vi "LinearSystemId_IdentifyDriveTrainSystem.vi"(8 "kAAngular":dbl, 9 "kVAngular":dbl, 10 "kALinear":dbl, 11 "kVLinear":dbl) -> (0 "Size Coerced":bool, 3 "Linearsystem":T1)   [LabVIEW 2019, in "Trajectory_Library.lvlib"]
doc: "Identify a standard differential drive drivetrain, given the drivetrain's kV and kA in both linear (volts/(meter/sec) and volts/(meter/sec^2)) and angular (volts/(meter/sec) and volts/(meter/sec^2)) cases. This can be found using frc-characterization. The linear system is defined as follows:\n\n - states\n - left velocity (m/s)\n - right velocity (m/s)\n - inputs\n - left voltage (volts)\n - right voltage(volts)\n - outputs\n - left velocity (m/s)\n - right velocity (m/s)\n\nInputs: \n - kVLinear -- The linear velocity gain, volts per (meter per second).\n - kALinear -- The linear acceleration gain, volts per (meter per second squared).\n - kVAngular -- The angular velocity gain, volts per (meter per second).\n - kAAngular -- The angular acceleration gain, volts per (meter per second squared).\n\nOutputs:\n - LinearSystem -- A LinearSystem representing the given characterized constants.\n - SizeCoerced -- A boolean indicating an error occured creating the system. A value of TRUE indicates an error.\n\nAdditional information\n https://github.com/wpilibsuite/frc-characterization"
uses:
  Trajectory_Library.lvlib
  TypeDef/LINEAR_SYSTEM.ctl
  <vilib>/Analysis/Matrix/Datatypes/RealMatrix.ctl
  MatrixHelper_CoerceSize.vi
  <vilib>/Analysis/Matrix/NI_Matrix.lvlib
panel:
  # "<States,States>"
  # "<States,Inputs>"
  # "<Outputs,States>"
  # "<Outputs,Inputs>"
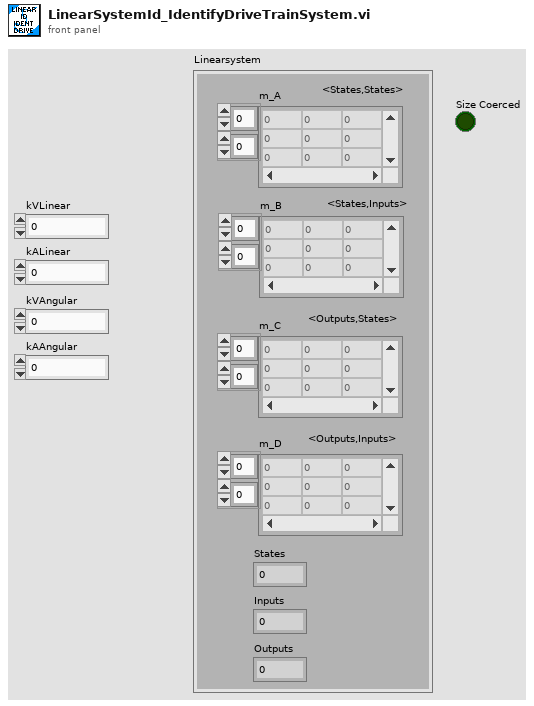
[diagram p1: front panel]
types:
  T1 = typedef "Trajectory_Library.lvlib/LINEAR_SYSTEM.ctl" = cluster{"m_A":T2, "m_B":T2, "m_C":T2, "m_D":T2, "States":i32, "Inputs":i32, "Outputs":i32}
  T2 = typedef "NI_Matrix.lvlib/RealMatrix.ctl" = dbl[][]
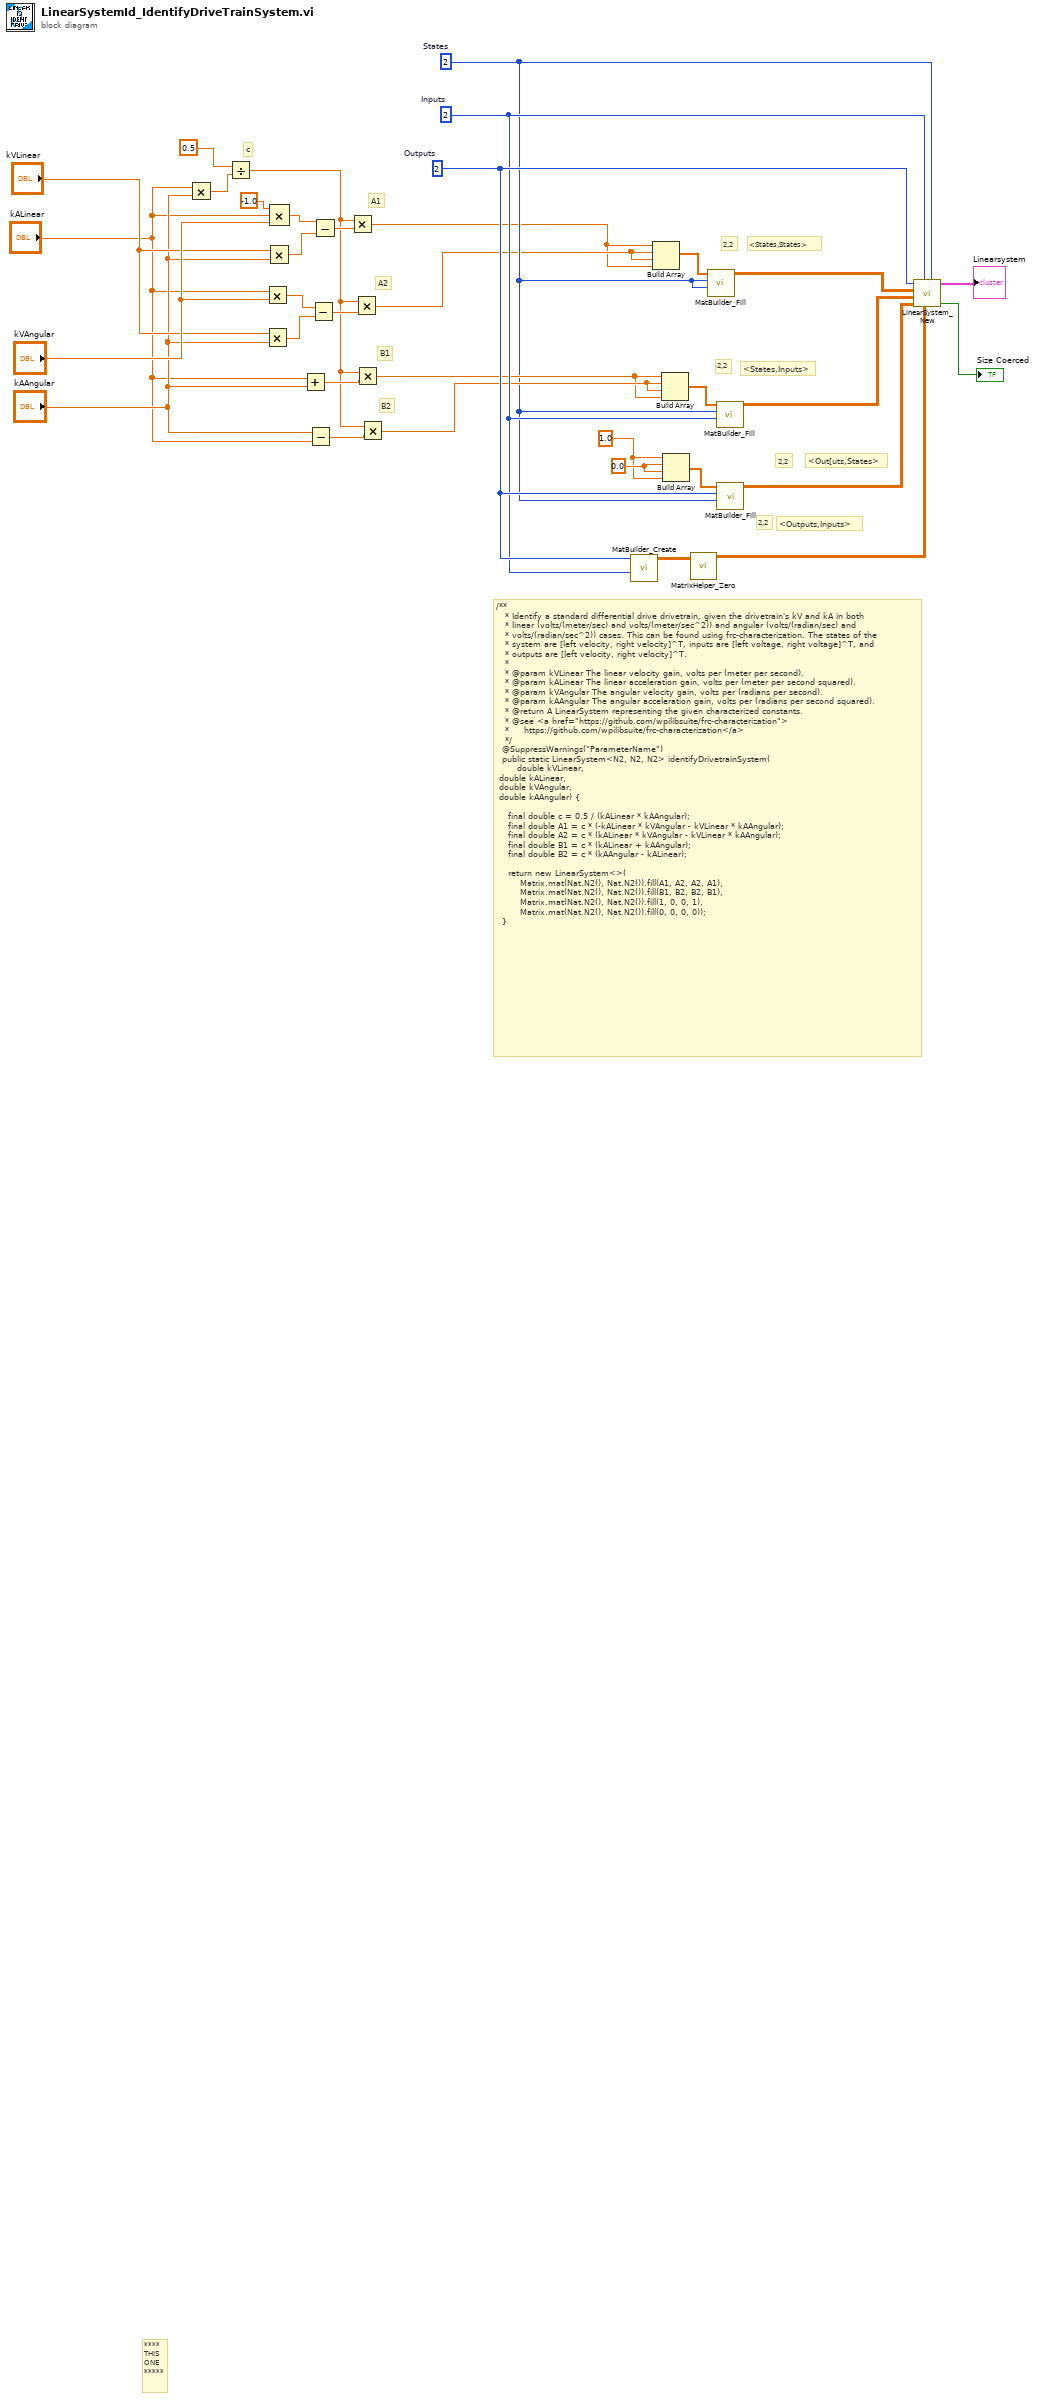
[diagram p0: block diagram]
diagram:
  w16 = 2  # Outputs
  w10 = 2  # Inputs
  w5 = 2  # States
  w15 = 0.0 ("element")
  w14 = 1.0 ("element")
  # "B2"
  # "B1"
  # "A2"
  # "A1"
  # "c"
  # "2,2"
  # "2,2"
  # "2,2"
  # "2,2"
  # "<States,States>"
  # "<States,Inputs>"
  # "<Out[uts,States>"
  # "<Outputs,Inputs>"
  # "/**\n   * Identify a standard differential drive drivetrain, given the drivetrain's kV and kA in both\n   * linear (volts/(meter/sec) and volts/(meter/sec^2)) and angular (volts/(radian/sec) and\n   * volts/(radian/sec^2)) cases. This can be found using frc-characterization. The states of the\n   * system are [left velocity, right velocity]^T, inputs are [left voltage, right voltage]^T, and\n   * outputs are [left velocity, right velocity]^T.\n   *\n   * @param kVLinear The linear velocity gain, volts per (meter per second).\n   * @param kALinear The linear acceleration gain, volts per (meter per second squared).\n   * @param kVAngular The angular velocity gain, volts per (radians per second).\n   * @param kAAngular The angular acceleration gain, volts per (radians per second squared).\n   * @return A LinearSystem representing the given characterized constants.\n   * @see <a href=\"https://github.com/wpilibsuite/frc-characterization\">\n   *     https://github.com/wpilibsuite/frc-characterization</a>\n   */\n  @SuppressWarnings(\"ParameterName\")\n  public static LinearSystem<N2, N2, N2> identifyDrivetrainSystem(\n      \tdouble kVLinear, \n\tdouble kALinear, \n\tdouble kVAngular, \n\tdouble kAAngular) {\n\n    final double c = 0.5 / (kALinear * kAAngular);\n    final double A1 = c * (-kALinear * kVAngular - kVLinear * kAAngular);\n    final double A2 = c * (kALinear * kVAngular - kVLinear * kAAngular);\n    final double B1 = c * (kALinear + kAAngular);\n    final double B2 = c * (kAAngular - kALinear);\n\n    return new LinearSystem<>(\n        Matrix.mat(Nat.N2(), Nat.N2()).fill(A1, A2, A2, A1),\n        Matrix.mat(Nat.N2(), Nat.N2()).fill(B1, B2, B2, B1),\n        Matrix.mat(Nat.N2(), Nat.N2()).fill(1, 0, 0, 1),\n        Matrix.mat(Nat.N2(), Nat.N2()).fill(0, 0, 0, 0));\n  }"
  # "****\nTHIS\nONE\n*****"
  n1 = Multiply(x="kALinear", y="kAAngular") -> (x*y=w33:dbl)
  n2 = Divide(x=0.5, y=w33) -> (x/y=w21:dbl)
  n3 = Multiply(x="kALinear", y="kVAngular") -> (x*y=w27:dbl)
  n4 = Multiply(x="kVLinear", y="kAAngular") -> (x*y=w28:dbl)
  n5 = Multiply(x="kVLinear", y="kAAngular") -> (x*y=w30:dbl)
  n6 = Compound Arithmetic op=MULTIPLY(-1.0 ("value"), "kALinear", "kVAngular") -> (w31:dbl)
  n7 = Add(x="kALinear", y="kAAngular") -> (x+y=w23:dbl)
  n8 = Subtract(x="kAAngular", y="kALinear") -> (x-y=w22:dbl)
  n9 = Subtract(x=w27, y=w28) -> (x-y=w26:dbl)
  n10 = Subtract(x=w31, y=w30) -> (x-y=w29:dbl)
  n11 = Multiply(x=w21, y=w29) -> (x*y=w2:dbl)
  n12 = Multiply(x=w21, y=w26) -> (x*y=w3:dbl)
  n13 = Multiply(x=w21, y=w23) -> (x*y=w7:dbl)
  n14 = Multiply(x=w21, y=w22) -> (x*y=w8:dbl)
  n15 = call "MatBuilder_Create.vi"("Columns"=w10, "Rows"=w16) -> ("output matrix"=w18:T2)  [unwired: 9 in]
  n16 = Build Array(w2, w3, w3, w2) -> (w4:dbl[])
  n17 = Build Array(w7, w8, w8, w7) -> (w9:dbl[])
  n18 = Build Array(w14, w15, w15, w14) -> (w13:dbl[])
  n19 = call "MatrixHelper_Zero.vi"("input matrix"=w18) -> ("output matrix"=w17:T2)  [unwired: 10 in]
  n20 = call "MatBuilder_Fill.vi"("Columns"=w5, "Rows"=w5, "Value List"=w4) -> ("output matrix"=w6:T2)  [unwired: 8 in]
  n21 = call "MatBuilder_Fill.vi"("Columns"=w10, "Rows"=w5, "Value List"=w9) -> ("output matrix"=w11:T2)  [unwired: 8 in]
  n22 = call "MatBuilder_Fill.vi"("Columns"=w5, "Rows"=w16, "Value List"=w13) -> ("output matrix"=w12:T2)  [unwired: 8 in]
  n23 = call "LinearSystem_New.vi"("States"=w5, "D"=w17, "Inputs"=w10, "C"=w12, "B"=w11, "A"=w6, "Outputs"=w16) -> ("Size Coerced"=→"Size Coerced":bool, "Linearsystem"=→"Linearsystem":T1)  [unwired: 3 in]
